vi "RAS RELAY 4.vi"(8 "entrée d'erreur (pas d'erreur)":errorcluster, 11 "LINX Resource en entrée":T1) -> (0 "sortie d'erreur":errorcluster, 3 "LINX Resource en sortie":T1)   [LabVIEW 2020]
uses:
  <vilib>/MakerHub/LINX/Private/Type Defs/LINX Ref.ctl
  <vilib>/MakerHub/LINX/Private/Type Defs/Platform.ctl
  <vilib>/MakerHub/LINX/Private/Type Defs/Interface.ctl
  <vilib>/MakerHub/LINX/Private/Device/Type Defs/LINX Device Config.ctl
  <vilib>/MakerHub/LINX/Private/Device/Type Defs/TCP Config.ctl
  <vilib>/MakerHub/LINX/Private/Device/Type Defs/Channels.ctl
  <vilib>/MakerHub/LINX/Public/Peripherals/Digital/Digital Write 1 Chan.vi
  <vilib>/MakerHub/LINX/Public/Peripherals/Digital/Digital Write N Chans.vi
  <vilib>/MakerHub/LINX/Private/Local IO/LinxDigitalWrite.vi
  <vilib>/MakerHub/LINX/Public/Utilities/Check Channel.vi
  <vilib>/MakerHub/LINX/Private/Utilties/Generate Error.vi
  <vilib>/MakerHub/LINX/LMH-LINX.lvlib
  <vilib>/MakerHub/LINX/Private/Device/Device.lvlib
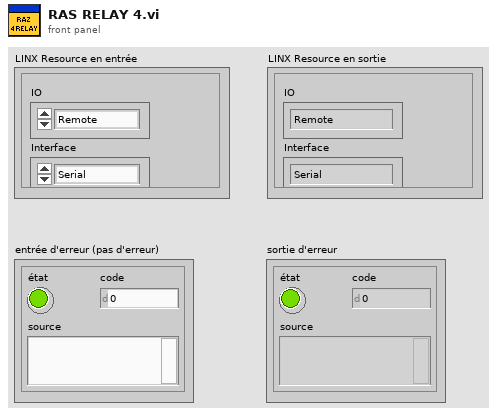
[diagram p1: front panel]
types:
  T1 = typedef "LMH-LINX.lvlib/LINX Ref.ctl" = cluster{"IO":T2, "Interface":T3, "LINX Device Config":T4}
  T2 = typedef "LMH-LINX.lvlib/Platform.ctl" = enum16{"Remote", "Local"}
  T3 = typedef "LMH-LINX.lvlib/Interface.ctl" = enum16{"Serial", "TCP"}
  T4 = typedef "LMH-LINX.lvlib/Device.lvlib/LINX Device Config.ctl" = cluster{"Interface":T3, "COM Port":refnum<visa-resource-name>, "TCP Configuration":T5, "Device Family":u8, "Device ID":u8, "Device Name":string, "TCP Ref":refnum<k5>, "Channels":T6}
  T5 = typedef "LMH-LINX.lvlib/Device.lvlib/TCP Config.ctl" = cluster{"IP Address":string, "Port":u16}
  T6 = typedef "LMH-LINX.lvlib/Channels.ctl" = cluster{"DI":u8[], "DO":u8[], "AI":u8[], "AO":u8[], "PWM":u8[], "QE":u8[], "UART":u8[], "I2C 2":u8[], "SPI":u8[], "CAN":u8[], "Servo":u8[], "AI Ref (V)":dbl, "AI Resolution (Bits)":u8, "AO Ref (V)":dbl, "AO Resolution (Bits)":u8}
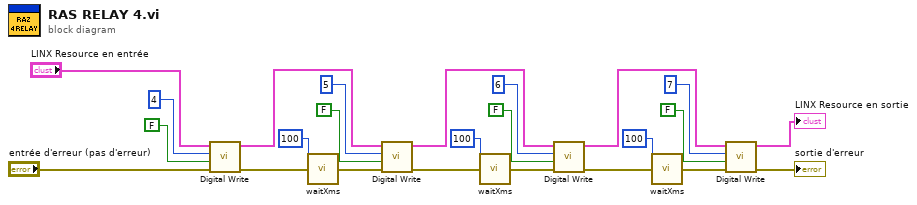
[diagram p0: block diagram]
diagram:
  n1 = call-poly <vilib>:"Digital Write.vi"("Error In"="entrée d'erreur (pas d'erreur)", "Output Value"=FALSE, "DO Channel"=u8 4, "LINX Resource"="LINX Resource en entrée") -> ("Error Out"=w19:errorcluster, "LINX Resource"=w24:T1)  [unwired: 6 in]
  n2 = call <userlib>:"waitXms.vi"("attente (ms)"=u32 100, "errin"=w19) -> ("errout"=w14:errorcluster)  [unwired: 13 in]
  n3 = call-poly <vilib>:"Digital Write.vi"("Error In"=w14, "Output Value"=FALSE, "DO Channel"=u8 5, "LINX Resource"=w24) -> ("Error Out"=w15:errorcluster, "LINX Resource"=w23:T1)  [unwired: 6 in]
  n4 = call <userlib>:"waitXms.vi"("attente (ms)"=u32 100, "errin"=w15) -> ("errout"=w13:errorcluster)  [unwired: 13 in]
  n5 = call-poly <vilib>:"Digital Write.vi"("Error In"=w13, "Output Value"=FALSE, "DO Channel"=u8 6, "LINX Resource"=w23) -> ("Error Out"=w12:errorcluster, "LINX Resource"=w22:T1)  [unwired: 6 in]
  n6 = call <userlib>:"waitXms.vi"("attente (ms)"=u32 100, "errin"=w12) -> ("errout"=w11:errorcluster)  [unwired: 13 in]
  n7 = call-poly <vilib>:"Digital Write.vi"("Error In"=w11, "Output Value"=FALSE, "DO Channel"=u8 7, "LINX Resource"=w22) -> ("Error Out"=→"sortie d'erreur":errorcluster, "LINX Resource"=→"LINX Resource en sortie":T1)  [unwired: 6 in]
